vi "LimitMotorPos.vi"(6 "Maximum pos":T2, 9 "max limit":T1, 10 "Min limit":T1, 11 "Position in":T2) -> (3 "Position out":T2)   [LabVIEW 2011]
uses:
  MotorPosType.ctl
  Typedefs/XYf.ctl
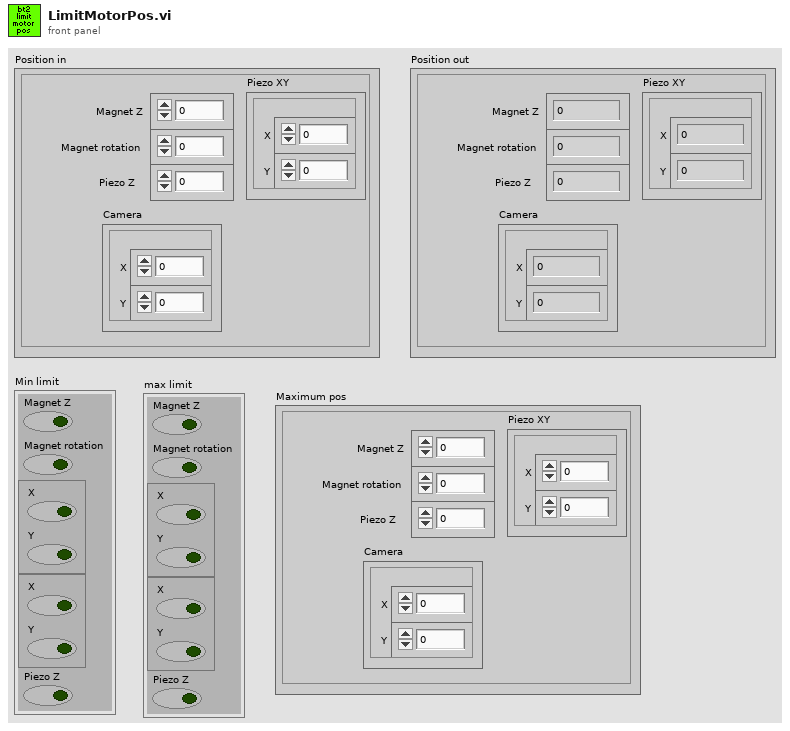
[diagram p1: front panel]
types:
  T1 = cluster{"Magnet Z":bool, "Magnet rotation":bool, cluster{"X":bool, "Y":bool}, cluster{"X":bool, "Y":bool}, "Piezo Z":bool}
  T2 = typedef "MotorPosType.ctl" = cluster{"Magnet Z":dbl, "Magnet rotation":dbl, "Camera":T3, "Piezo XY":T3, "Piezo Z":dbl}
  T3 = typedef "XYf.ctl" = cluster{"X":sgl, "Y":sgl}
  T4 = cluster{"Magnet Z":bool, "Magnet rotation":bool, "Camera":cluster{"X":bool, "Y":bool}, "Piezo XY":cluster{"X":bool, "Y":bool}, "Piezo Z":bool}
  T5 = cluster{"Magnet Z":i16, "Magnet rotation":i16, cluster{"X":i16, "Y":i16}, cluster{"X":i16, "Y":i16}, "Piezo Z":i16}
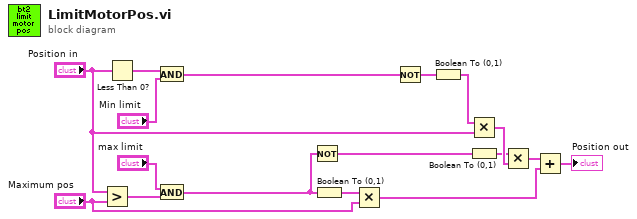
[diagram p0: block diagram]
diagram:
  n1 = Greater?(x="Position in", y="Maximum pos") -> (0:w4:T4)
  n2 = Less Than 0?(x="Position in") -> (x < 0?=w1:T1)
  n3 = And(x=w1, y="Min limit") -> (x .and. y?=w6:T1)
  n4 = And(x="max limit", y=w4) -> (x .and. y?=w8:T1)
  n5 = Not(x=w8) -> (.not. x?=w9:T1)
  n6 = Boolean To (0,1)(Boolean=w8) -> (0, 1=w10:T5)
  n7 = Multiply(x=w10, y="Maximum pos") -> (x*y=w15:T2)
  n8 = Not(x=w6) -> (.not. x?=w7:T1)
  n9 = Boolean To (0,1)(Boolean=w7) -> (0, 1=w5:T5)
  n10 = Multiply(x=w5, y="Position in") -> (x*y=w14:T2)
  n11 = Boolean To (0,1)(Boolean=w9) -> (0, 1=w11:T5)
  n12 = Multiply(x=w11, y=w14) -> (x*y=w16:T2)
  n13 = Add(x=w16, y=w15) -> (x+y=→"Position out":T2)
